vi "Main.vi"() -> ()   [LabVIEW 2016, in "Utilities.lvlib" / "Simple Counter.lvlib"]
uses:
  Simple Counter.lvlib
  States.ctl
  Data.ctl
  Drivers/C8855-01/Transfer Mode.ctl
  Drivers/C8855-01/C8855-01.lvlib
panel:
  in  "Quit":bool
  out "ID":string
  out "Counts":i32 format="%d cps"
  out "History":i32(graph)
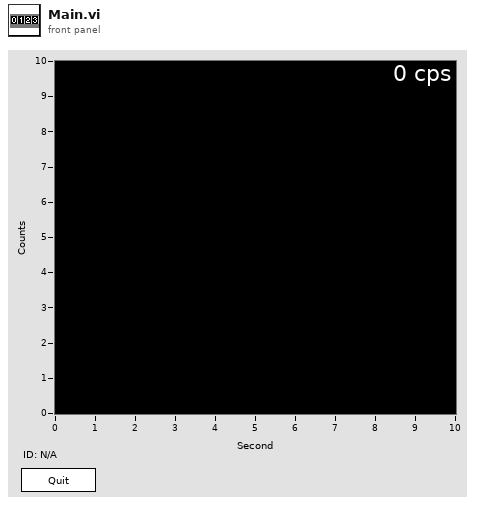
[diagram p1: front panel]
types:
  T1 = typedef "Utilities.lvlib/Simple Counter.lvlib/Data.ctl" = cluster{"Handle":u32, "Buffer":u16[]}
  T2 = typedef "Utilities.lvlib/Simple Counter.lvlib/States.ctl" = enum16{"Init", "Open", "Setup", "Idle", "Error", "Close", "Clear", "Exit"}
  T3 = typedef "Drivers.lvlib/C8855-01.lvlib/Transfer Mode.ctl" = u8
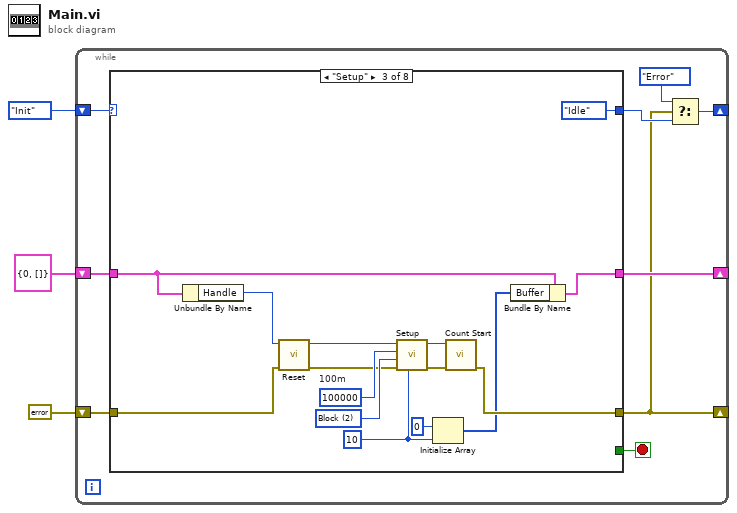
[diagram p0: block diagram]
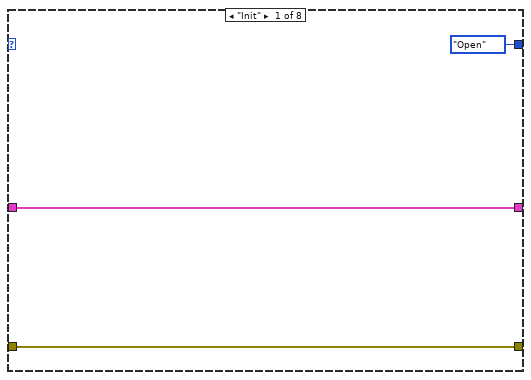
[diagram p2: hidden frame]
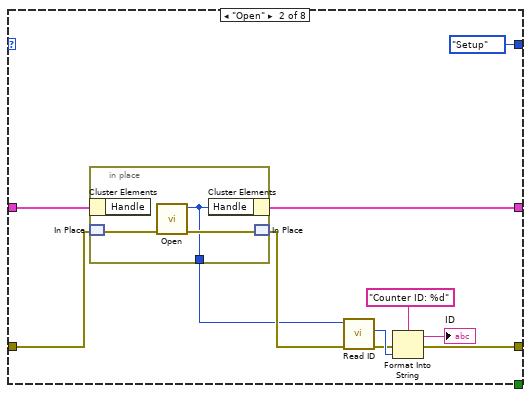
[diagram p3: hidden frame]
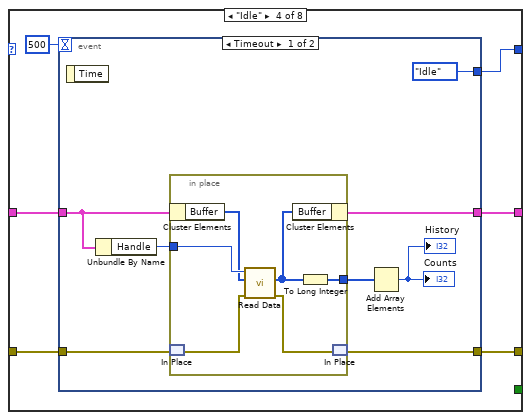
[diagram p4: hidden frame]
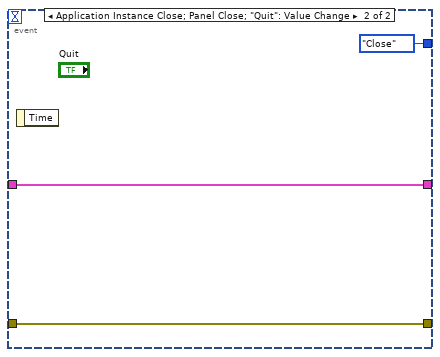
[diagram p5: hidden frame]
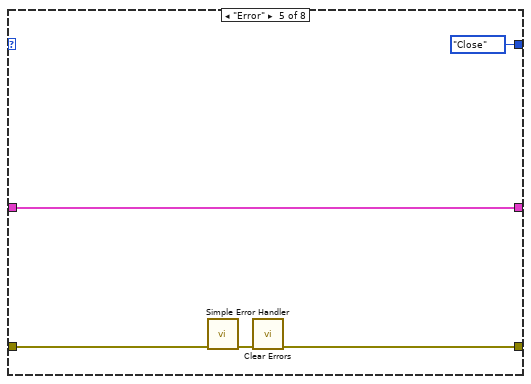
[diagram p6: hidden frame]
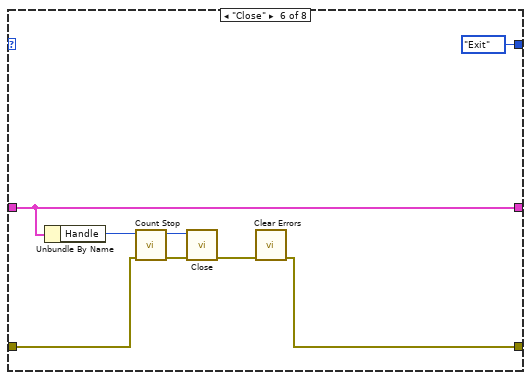
[diagram p7: hidden frame]
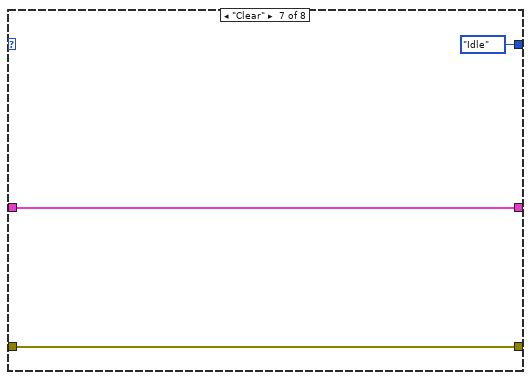
[diagram p8: hidden frame]
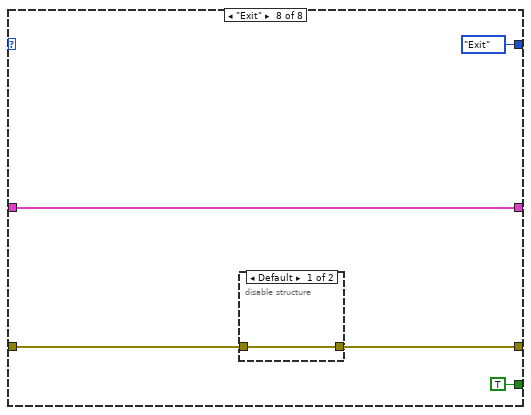
[diagram p9: hidden frame]
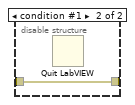
[diagram p10: hidden frame]
diagram:
  n1 = while {
    shift-right: [w4] -> _
    shift-left: States."Init" -> [w11]
    shift-right: [w6] -> _
    shift-left: errorcluster {"status"=FALSE, "code"=0, "source"=""} ("error in (no error)") -> [w10]
    shift-right: [w8] -> _
    shift-left: T1 {"Handle"=0, "Buffer"=[]} -> [w9]
    stop <- w12 stop-if-true
    n2 = case shown="\"Setup\"" w11 {
      tunnel: [_ _ _ _ _ _ _ TRUE] -> w12
      tunnel: [States."Open" States."Setup" States."Idle" w46 States."Close" States."Exit" States."Idle" States."Exit"] -> w7
      tunnel: w10 -> [w14 w23 w35 w50 w71 w75 w81 w84]
      tunnel: w9 -> [w13 w25 w34 w47 w72 w79 w82 w86]
      tunnel: [w13 w24 w33 w48 w72 w79 w82 w86] -> w8
      tunnel: [w14 w16 w39 w49 w69 w73 w81 w85] -> w6
      frame "Init" {
      }
      frame "Open" {
        n3 = in-place {
          in-place-border: [w27] -> w21
          n4 = in-place-cluster #1(w25) -> ()  [unwired: 1 out]
          n5 = in-place-match #2(w23) -> (w28:errorcluster)
          n6 = call "Open.vi"("error in (no error)"=w28) -> ("error out"=w29:errorcluster, "Handle"=w27:u32)  [unwired: 9 in]
          n7 = in-place-cluster #1("Handle"=w27) -> (w24:T1)
          n8 = in-place-match #2(w29) -> (w22:errorcluster)
        }
        n9 = call "Read ID.vi"("error in (no error)"=w22, "handle in"=w21) -> ("error out"=w17:errorcluster, "ID"=w19:u8)  [unwired: 7 in, 1 out]
        n10 = Format Into String(format string="Counter ID: %d", error in=w17, w19) -> (resulting string=→"ID":string, error out=w16:errorcluster)  [unwired: 1 in]
      }
      frame "Setup" {
        w32 = u16 10 ("Number of Gate")
        w43 = u32 100000  # 100m
        w42 = T3 2 items=["Single"=1, "Block"=2] ("Transfer Mode")
        n11 = Unbundle By Name(w34) -> ("Handle"=w37:u32)
        n12 = call "Reset.vi"("error in (no error)"=w35, "handle in"=w37) -> ("error out"=w38:errorcluster, "handle out"=w36:u32)  [unwired: 8 in]
        n13 = call "Setup.vi"("Number of Gate"=w32, "error in (no error)"=w38, "Transfer Mode"=w42, "Gate Time (us)"=w43, "Handle"=w36) -> ("error out"=w40:errorcluster, "Handle out"=w41:u32)  [unwired: 5 in]
        n14 = Initialize Array(u16 0 ("element"), w32) -> (w30:u16[])
        n15 = call "Count Start.vi"("error in (no error)"=w40, "handle in"=w41) -> ("error out"=w39:errorcluster)  [unwired: 8 in, 1 out]
        n16 = Bundle By Name(cluster=w34, "Buffer"=w30) -> (w33:T1)
      }
      frame "Idle" {
        n17 = event shown="[0] Timeout" {
          selector: _ -> [_ _]
          dyn-events: _ -> [_ _]
          timeout: 500 -> [_ _]
          tunnel: w50 -> [w52 w65]
          tunnel: [w51 w65] -> w49
          tunnel: [w53 w66] -> w48
          tunnel: w47 -> [w54 w66]
          tunnel: [States."Idle" States."Close"] -> w46
          event Timeout {
            n18 = event-data() -> ()  [unwired: 1 in, 1 out]
            n19 = Unbundle By Name(w54) -> ("Handle"=w57:u32)
            n20 = in-place {
              in-place-border: w57 -> [w64]
              in-place-border: [w63] -> w55
              n21 = in-place-cluster #3(w54) -> ("Buffer"=w60:u16[])
              n22 = in-place-match #4(w52) -> (w62:errorcluster)
              n23 = call "Read Data.vi"("error in (no error)"=w62, "buffer in"=w60, "handle in"=w64) -> ("error out"=w61:errorcluster, "buffer out"=w59:u16[])  [unwired: 6 in, 1 out]
              n24 = in-place-cluster #3("Buffer"=w59) -> (w53:T1)
              n25 = To Long Integer(number=w59) -> (32bit integer=w63:i32[])
              n26 = in-place-match #4(w61) -> (w51:errorcluster)
            }
            n27 = Add Array Elements(numeric array=w55) -> (sum=→"History" →"Counts":i32)
          }
          event Application Instance Close; Panel Close; "Quit": Value Change {
            n28 = event-data() -> ()  [unwired: 1 in, 1 out]
          }
        }
      }
      frame "Error" {
        n29 = call <vilib>:"Simple Error Handler.vi"("error in (no error)"=w71) -> ("error out"=w70:errorcluster)  [unwired: 4 in, 4 out]
        n30 = call <vilib>:"Clear Errors.vi"("error in (no error)"=w70) -> ("error out"=w69:errorcluster)  [unwired: 5 in, 1 out]
      }
      frame "Close" {
        n31 = Unbundle By Name(w79) -> ("Handle"=w78:u32)
        n32 = call "Count Stop.vi"("error in (no error)"=w75, "handle in"=w78) -> ("error out"=w76:errorcluster, "handle out"=w77:u32)  [unwired: 8 in]
        n33 = call "Close.vi"("error in (no error)"=w76, "handle in"=w77) -> ("error out"=w74:errorcluster)  [unwired: 9 in]
        n34 = call <vilib>:"Clear Errors.vi"("error in (no error)"=w74) -> ("error out"=w73:errorcluster)  [unwired: 5 in, 1 out]
      }
      frame "Clear" {
      }
      frame "Exit" {
        n35 = disable-structure shown="Default" {
          disable-tunnel: [w89 w90] -> w85
          disable-tunnel: w84 -> [w89 w90]
          frame condition #0 (active) {
          }
          frame condition #1 {
            n36 = Quit LabVIEW() -> ()  [unwired: 1 in]
          }
        }
      }
    }
    n37 = Select(t=States."Error", s=w6, f=w7) -> (s? t:f=w4:T2)
  }
